vi "Parse Generic Socket CAN.vi"(10 "Bytes in":u8[](array[numeric]), 11 "pcap Parse and Build in":refnum<class "pcap_Parse_Build_CIF.lvclass">) -> (0 "ID":u32 format="%.0x", 1 "FD Flags":u8 format="%.0x", 2 "Payload":u8[](array[numeric]) format="%.0x", 3 "pcap Parse and Build out":refnum<class "pcap_Parse_Build_CIF.lvclass">, 4 "Remote":bool, 5 "Extended":bool, 6 "TAI Time (ns)":i64)   [LabVIEW 2021, in "pcap_Parse_Build_CIF.lvclass"]
uses:
  pcap_Parse_Build_CIF.lvclass
  pcap_Parse_Build_CIF.lvclass/pcap_Parse_Build_CIF.ctl
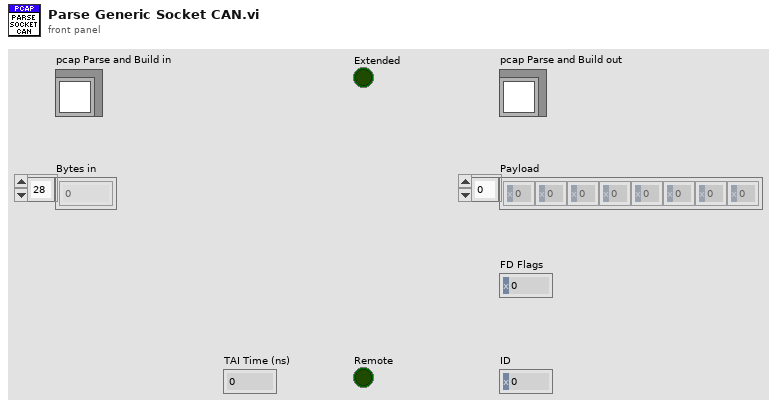
[diagram p1: front panel]
types:
  T1 = typedef "pcap_Parse_Build_CIF.lvclass/Socket CAN Header.ctl" = cluster{"CANID and Flags":u32, "Payload Length":u8, "FD Flags":u8, "RSVD":u8, "Len8 DLC":u8}
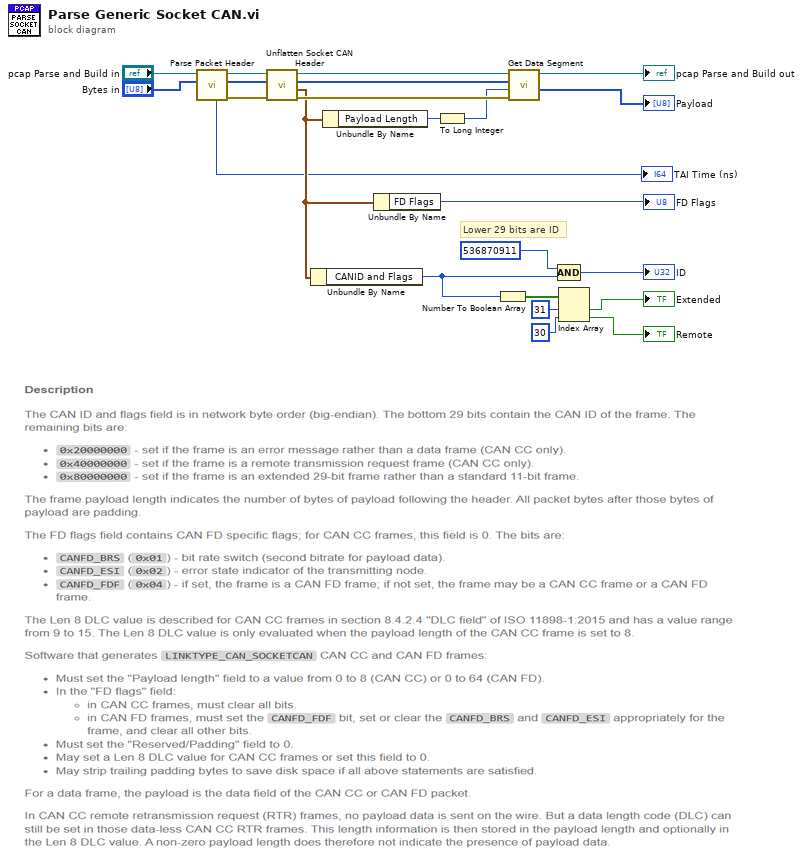
[diagram p0: block diagram]
diagram:
  # "Lower 29 bits are ID"
  n1 = call "Parse Packet Header.vi"("Bytes in"="Bytes in", "pcap Parse and Build in"="pcap Parse and Build in") -> ("error out"=w12:errorcluster, "Bytes out"=w13:u8[], "pcap Parse and Build out"=w14:refnum<class "pcap_Parse_Build_CIF.lvclass">, "TAI Time (ns)"=→"TAI Time (ns)":i64)  [unwired: 4 in, 2 out]
  n2 = call "Unflatten Socket CAN Header.vi"("error in (no error)"=w12, "Bytes in"=w13, "pcap Parse and Build in"=w14) -> ("error out"=w9:errorcluster, "Socket CAN Header"=w3:T1, "Bytes out"=w10:u8[], "pcap Parse and Build out"=w11:refnum<class "pcap_Parse_Build_CIF.lvclass">)  [unwired: 5 in]
  n3 = Unbundle By Name(w3) -> ("CANID and Flags"=w21:u32)
  n4 = Unbundle By Name(w3) -> ("Payload Length"=w8:u8)
  n5 = Unbundle By Name(w3) -> ("FD Flags"=→"FD Flags":u8)
  n6 = To Long Integer(number=w8) -> (32bit integer=w7:i32)
  n7 = Number To Boolean Array(number=w21) -> (Boolean array=w20:bool[])
  n8 = call "Get Data Segment.vi"("error in (no error)"=w9, "Length"=w7, "Bytes in"=w10, "pcap Parse and Build in"=w11) -> ("Data Segment"=→"Payload":u8[], "pcap Parse and Build out"=→"pcap Parse and Build out":refnum<class "pcap_Parse_Build_CIF.lvclass">)  [unwired: 4 in, 2 out]
  n9 = Compound Arithmetic op=AND(u32 536870911 ("number"), w21) -> (→"ID":u32)
  n10 = Index Array(array=w20, index #1=31 ("index"), index #2=30 ("index")) -> (element #1=→"Extended":bool, element #2=→"Remote":bool)
